vi "example-VINameToVI.vi"() -> ()   [LabVIEW 2019]
uses:
  SetGetControlValue.lvlib
panel:
  out "Values":string[](array[string])
  in  "VI Name":string
  in  "Control Names":string[](array[string])
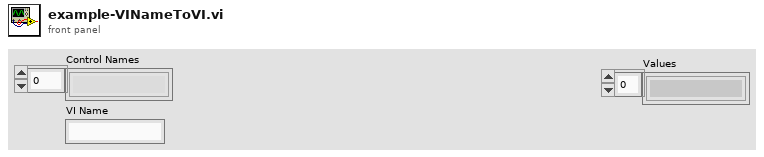
[diagram p1: front panel]
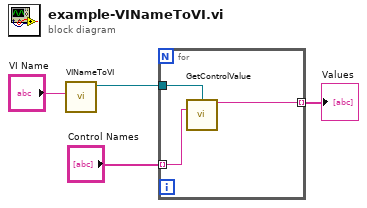
[diagram p0: block diagram]
diagram:
  n1 = call "VINameToVI.vi"("vi"="VI Name") -> ("VI out"=w2:refnum<vi>)  [unwired: 9 in, 1 out]
  n2 = for {
    tunnel: "Control Names" -> [w7] mode=indexing
    tunnel: w2 -> [w6]
    tunnel: [w5] -> w1 mode=indexing
    n3 = call "GetControlValue.vi"("vi ref"=w6, "ctrl"=w7) -> ("String out"=w5:string)  [unwired: 11 in, 2 out]
  }
  "Values" <- w1
